vi "Test 2.vi"() -> ()   [LabVIEW 2012, in "Universal Power Meter.lvlib"]
uses:
  Universal Power Meter.lvlib
  Universal Power Meter.lvclass
  Generic Instrument/Generic Instrument.lvclass
  Yokogawa WT2X0/Yokogawa WT2X0.lvclass
panel:
  in  "Option":string
  out "Power Meter Visa":refnum<visa-resource-name>
  out "Model":string
  out "String":string
  out "f":dbl
  in  "ID cluster.Model":string
  in  "Number of Cards":dbl
  in  "THD?":bool
  in  "ID":string
  out "Yokogawa WT2X0 out":refnum<class "Yokogawa WT2X0.lvclass">
  in  "Yokogawa WT2X0 in":refnum<class "Yokogawa WT2X0.lvclass">
  out "error out":errorcluster
  in  "error in (no error)":errorcluster
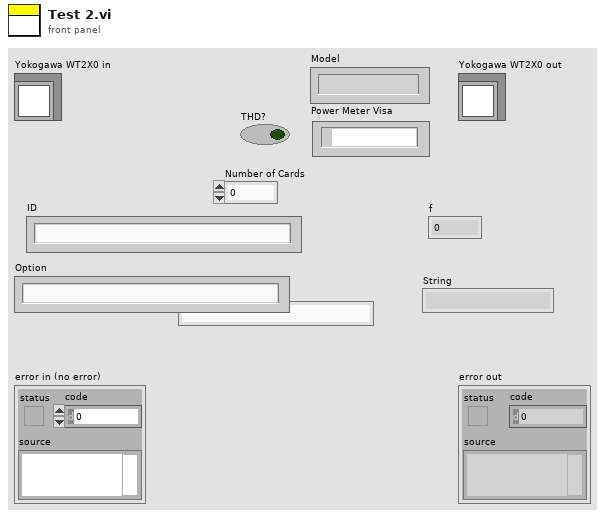
[diagram p1: front panel]
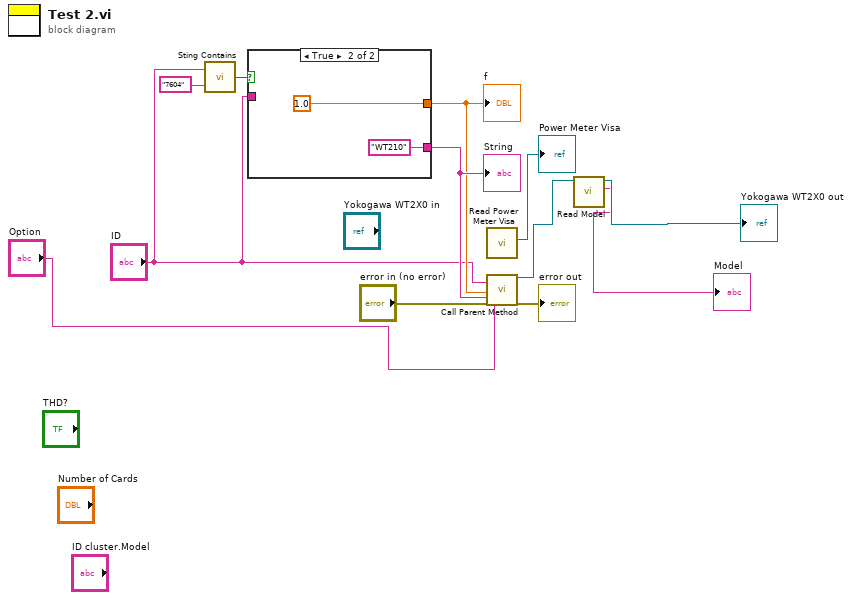
[diagram p0: block diagram]
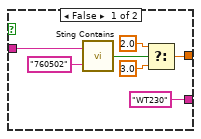
[diagram p2: hidden frame]
diagram:
  n1 = call "Sting Contains.vi"("Expression to evaluate"="7604", "Input String"="ID") -> ("Boolean"=w9:bool)
  n2 = case shown="True" w9 {
    tunnel: [w14 1.0] -> w7
    tunnel: "ID" -> [w19 _]
    tunnel: ["WT230" "WT210"] -> w8
    frame False {
      n3 = call "Sting Contains.vi"("Expression to evaluate"="760502", "Input String"=w19) -> ("Boolean"=w17:bool)
      n4 = Select(t=2.0, s=w17, f=3.0) -> (s? t:f=w14:dbl)
    }
    frame True {
    }
  }
  "f" <- w7
  "String" <- w8
  n5 = call "Read Power Meter Visa.vi"() -> ("Power Meter Visa"=→"Power Meter Visa":refnum<visa-resource-name>)  [unwired: 9 in, 2 out]
  n6 = call-parent "Call Parent Method"("ID"="ID", "Number of Cards"=w7, "ID cluster.Model"=w8, "error in (no error)"="error in (no error)", "Option"="Option") -> ("Universal Power Meter out"=w3:refnum<class "Yokogawa WT2X0.lvclass">, "error out"=→"error out":errorcluster)  [unwired: 13 in]
  n7 = call "Read Model.vi"("Generic Instrument in"=w3) -> ("Model"=→"Model":string, "Generic Instrument out"=→"Yokogawa WT2X0 out":refnum<class "Yokogawa WT2X0.lvclass">)  [unwired: 8 in, 1 out]
